vi "Helmholtz2D_FEM_Polyarea.vi"(10 "Y":dbl[](array[numeric]), 11 "X":dbl[](array[numeric])) -> (3 "area":dbl)   [LabVIEW 2020, in "NI_PDE.lvlib"]
uses:
  <vilib>/gmath/NI_PDE.lvlib
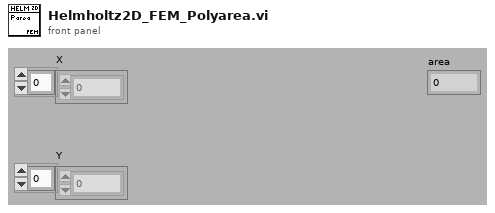
[diagram p1: front panel]
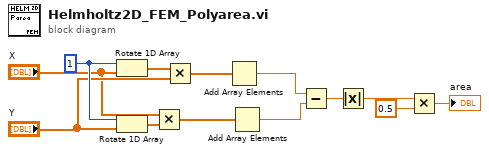
[diagram p0: block diagram]
diagram:
  w10 = 1 ("n")
  n1 = Rotate 1D Array(1:"X", 2:w10) -> (0:w8:dbl[])
  n2 = Rotate 1D Array(1:"Y", 2:w10) -> (0:w3:dbl[])
  n3 = Multiply(x="X", y=w3) -> (x*y=w2:dbl[])
  n4 = Multiply(x=w8, y="Y") -> (x*y=w6:dbl[])
  n5 = Add Array Elements(numeric array=w6) -> (sum=w5:dbl)
  n6 = Add Array Elements(numeric array=w2) -> (sum=w1:dbl)
  n7 = Subtract(x=w5, y=w1) -> (x-y=w13:dbl)
  n8 = Absolute Value(x=w13) -> (abs(x)=w12:dbl)
  n9 = Multiply(x=w12, y=0.5) -> (x*y=→"area":dbl)
